vi "Serial Port Selection Tester 2012 NIVerified.vi"() -> ()   [LabVIEW 2012]
panel:
  out "VISA resource name out":refnum<visa-resource-name>
  # "Overview: Allows the user to manually select which serial port they would like to use in their program.\nRequirement:\nSoftware:\n    Labview 2012 (or compatible)\nHardware:\n    USB-232 device \nInstructions:\n1. Ensure USB-232 device is normally connected\n2. Run the VI"
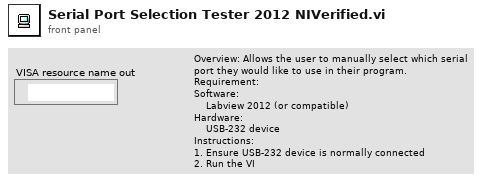
[diagram p1: front panel]
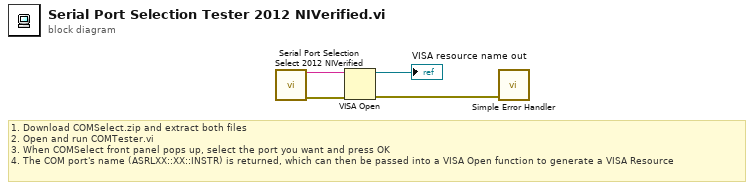
[diagram p0: block diagram]
diagram:
  # "1. Download COMSelect.zip and extract both files\n2. Open and run COMTester.vi\n3. When COMSelect front panel pops up, select the port you want and press OK\n4. The COM port's name (ASRLXX::XX::INSTR) is returned, which can then be passed into a VISA Open function to generate a VISA Resource"
  n1 = call "Serial Port Selection Select 2012 NIVerified.vi"() -> ("error out"=w3:errorcluster, "COM Port Selected"=w4:string)  [unwired: 1 in, 8 out]
  n2 = VISA Open(error in (no error)=w3, VISA resource name=w4) -> (VISA resource name=→"VISA resource name out":refnum<visa-resource-name>, error out=w1:errorcluster)  [unwired: 3 out]
  n3 = call <vilib>:"Simple Error Handler.vi"("error in (no error)"=w1) -> ()  [unwired: 4 in, 5 out]
